vi "Read instances allowed.vi"(8 "error in":errorcluster, 11 "DecideProjectFeatures in":refnum<class "DCAFConfigurablePluginDecideFeatures.lvclass">) -> (0 "error out":errorcluster, 2 "instances allowed":i32, 3 "DecideProjectFeatures out":refnum<class "DCAFConfigurablePluginDecideFeatures.lvclass">)   [LabVIEW 2013, in "DCAFConfigurablePluginDecideFeatures.lvclass"]
uses:
  DCAFConfigurablePluginDecideFeatures.lvclass
  DCAFConfigurablePluginDecideFeatures.lvclass/DCAFConfigurablePluginDecideFeatures.ctl
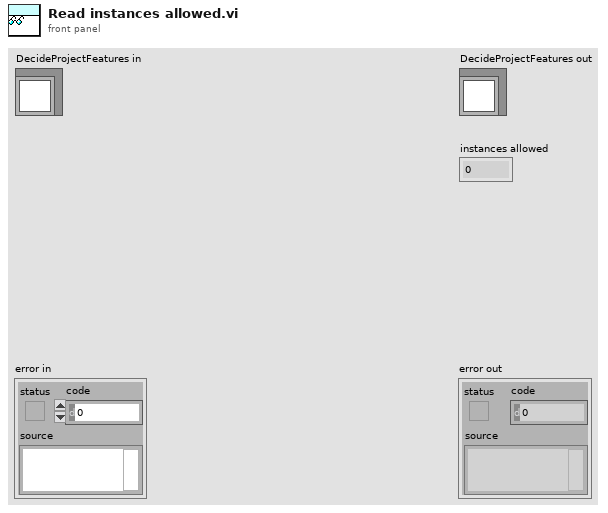
[diagram p1: front panel]
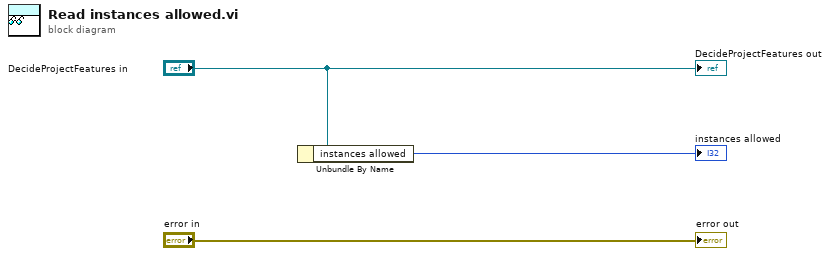
[diagram p0: block diagram]
diagram:
  n1 = Unbundle By Name("DecideProjectFeatures in") -> ("instances allowed"=→"instances allowed":i32)
  "error out" <- "error in"
  "DecideProjectFeatures out" <- "DecideProjectFeatures in"
